vi "Agilent 34970 Temperature Resistance Conversion.vi"(6 "Resistance Value":dbl, 8 "error in (no error)":errorcluster) -> (0 "error out":errorcluster, 4 "Temperature (F)":dbl)   [LabVIEW 2023]
uses:
  <vilib>/Analysis/NI_AALPro.lvlib
panel:
  out "Temperature (C)":dbl
  out "Temperature Array":dbl[](array[numeric])
  out "Resistance Array":dbl[](array[numeric])
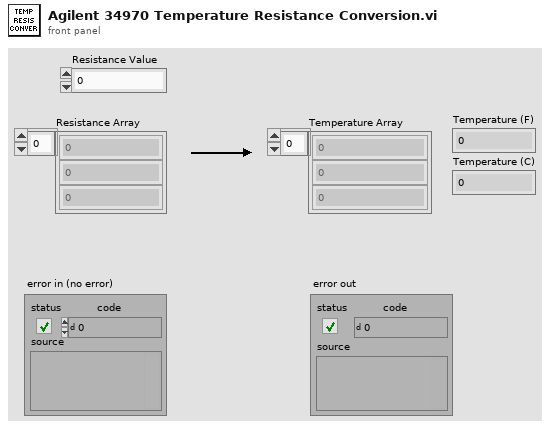
[diagram p1: front panel]
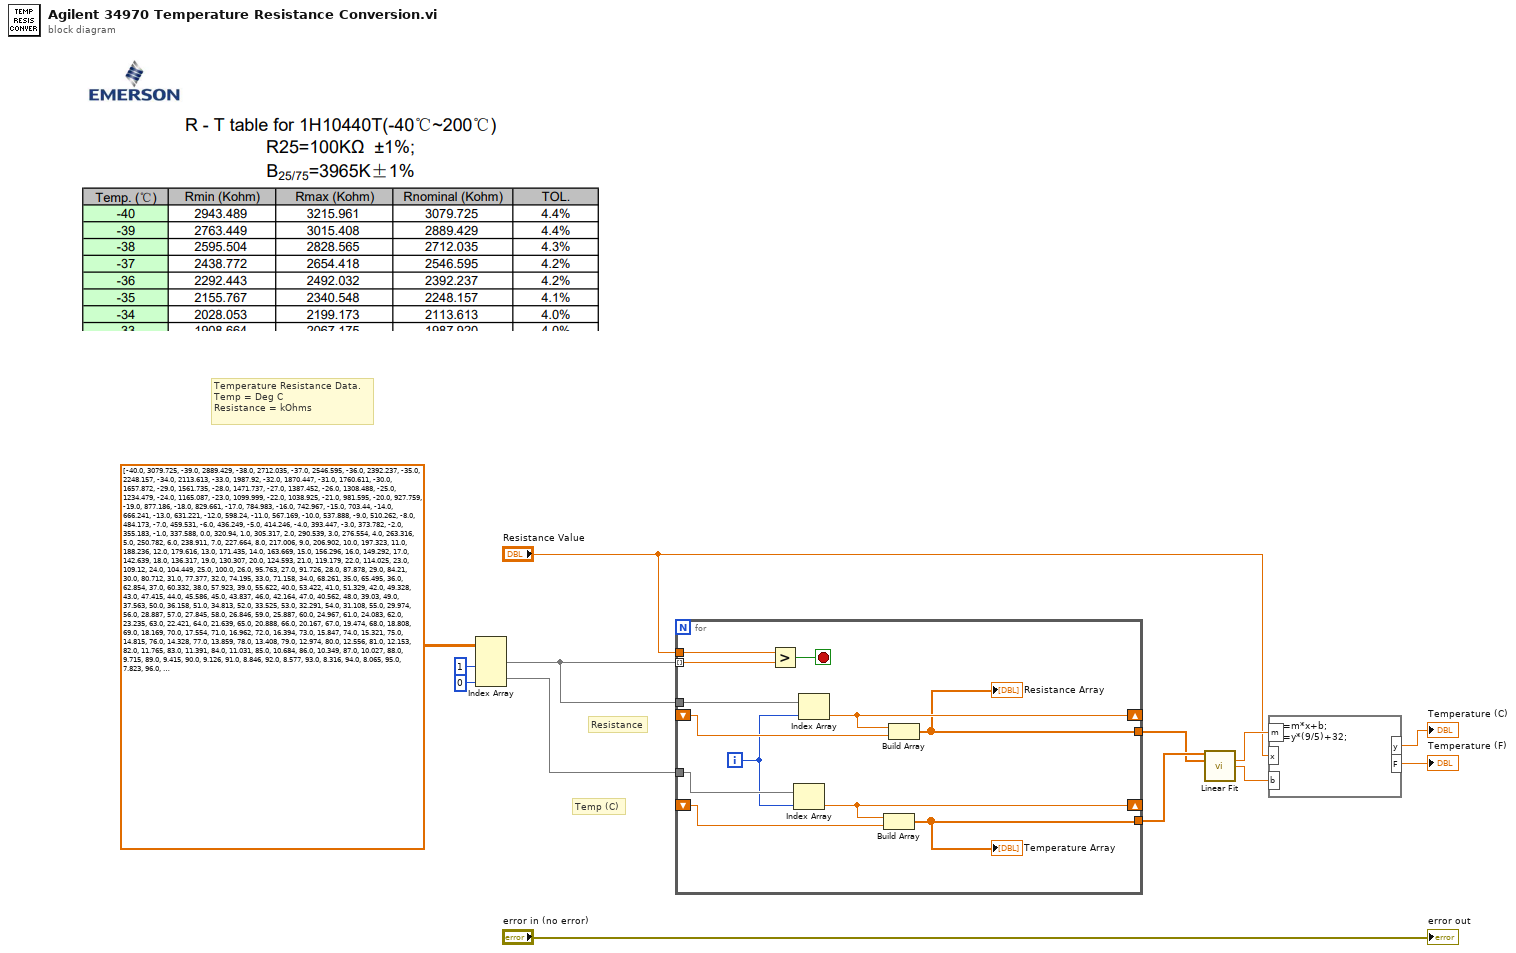
[diagram p0: block diagram]
diagram:
  # "Temp (C)"
  # "Resistance"
  # "Temperature Resistance Data. \nTemp = Deg C\nResistance = kOhms"
  n1 = Index Array(array=dbl[][] [[-40.0, 3079.725], [-39.0, 2889.429], [-38.0, 2712.035], [-37.0, 2546.595], [-36.0, 2392.237], [-35.0, 2248.157], [-34.0, 2113.613], [-33.0, 1987.92], [-32.0, 1870.447], [-31.0, 1760.611], [-30.0, 1657.872], [-29.0, 1561.735], [-28.0, 1471.737], [-27.0, 1387.452], [-26.0, 1308.488], [-25.0, 1234.479], [-24.0, 1165.087], [-23.0, 1099.999], [-22.0, 1038.925], [-21.0, 981.595], [-20.0, 927.759], [-19.0, 877.186], [-18.0, 829.661], [-17.0, 784.983], [-16.0, 742.967], [-15.0, 703.44], [-14.0, 666.241], [-13.0, 631.221], [-12.0, 598.24], [-11.0, 567.169], [-10.0, 537.888], [-9.0, 510.262], [-8.0, 484.173], [-7.0, 459.531], [-6.0, 436.249], [-5.0, 414.246], [-4.0, 393.447], [-3.0, 373.782], [-2.0, 355.183], [-1.0, 337.588], [0.0, 320.94], [1.0, 305.317], [2.0, 290.539], [3.0, 276.554], [4.0, 263.316], [5.0, 250.782], [6.0, 238.911], [7.0, 227.664], [8.0, 217.006], [9.0, 206.902], [10.0, 197.323], [11.0, 188.236], [12.0, 179.616], [13.0, 171.435], [14.0, 163.669], [15.0, 156.296], [16.0, 149.292], [17.0, 142.639], [18.0, 136.317], [19.0, 130.307], [20.0, 124.593], [21.0, 119.179], [22.0, 114.025], [23.0, 109.12], [24.0, 104.449], [25.0, 100.0], [26.0, 95.763], [27.0, 91.726], [28.0, 87.878], [29.0, 84.21], [30.0, 80.712], [31.0, 77.377], [32.0, 74.195], [33.0, 71.158], [34.0, 68.261], [35.0, 65.495], [36.0, 62.854], [37.0, 60.332], [38.0, 57.923], [39.0, 55.622], [40.0, 53.422], [41.0, 51.329], [42.0, 49.328], [43.0, 47.415], [44.0, 45.586], [45.0, 43.837], [46.0, 42.164], [47.0, 40.562], [48.0, 39.03], [49.0, 37.563], [50.0, 36.158], [51.0, 34.813], [52.0, 33.525], [53.0, 32.291], [54.0, 31.108], [55.0, 29.974], [56.0, 28.887], [57.0, 27.845], [58.0, 26.846], [59.0, 25.887], [60.0, 24.967], [61.0, 24.083], [62.0, 23.235], [63.0, 22.421], [64.0, 21.639], [65.0, 20.888], [66.0, 20.167], [67.0, 19.474], [68.0, 18.808], [69.0, 18.169], [70.0, 17.554], [71.0, 16.962], [72.0, 16.394], [73.0, 15.847], [74.0, 15.321], [75.0, 14.815], [76.0, 14.328], [77.0, 13.859], [78.0, 13.408], [79.0, 12.974], [80.0, 12.556], [81.0, 12.153], [82.0, 11.765], [83.0, 11.391], [84.0, 11.031], [85.0, 10.684], [86.0, 10.349], [87.0, 10.027], [88.0, 9.715], [89.0, 9.415], [90.0, 9.126], [91.0, 8.846], [92.0, 8.577], [93.0, 8.316], [94.0, 8.065], [95.0, 7.823], [96.0, 7.589], [97.0, 7.363], [98.0, 7.144], [99.0, 6.933], [100.0, 6.73], [101.0, 6.534], [102.0, 6.344], [103.0, 6.161], [104.0, 5.984], [105.0, 5.812], [106.0, 5.646], [107.0, 5.486], [108.0, 5.331], [109.0, 5.181], [110.0, 5.035], [111.0, 4.894], [112.0, 4.758], [113.0, 4.626], [114.0, 4.499], [115.0, 4.375], [116.0, 4.255], [117.0, 4.139], [118.0, 4.027], [119.0, 3.918], [120.0, 3.812], [121.0, 3.71], [122.0, 3.612], [123.0, 3.516], [124.0, 3.423], [125.0, 3.333], [126.0, 3.246], [127.0, 3.162], [128.0, 3.08], [129.0, 3.0], [130.0, 2.923], [131.0, 2.848], [132.0, 2.775], [133.0, 2.705], [134.0, 2.636], [135.0, 2.57], [136.0, 2.505], [137.0, 2.442], [138.0, 2.382], [139.0, 2.322], [140.0, 2.265], [141.0, 2.209], [142.0, 2.155], [143.0, 2.102], [144.0, 2.051], [145.0, 2.001], [146.0, 1.953], [147.0, 1.906], [148.0, 1.86], [149.0, 1.815], [150.0, 1.772], [151.0, 1.73], [152.0, 1.689], [153.0, 1.65], [154.0, 1.611], [155.0, 1.573], [156.0, 1.537], [157.0, 1.501], [158.0, 1.467], [159.0, 1.433], [160.0, 1.401], [161.0, 1.369], [162.0, 1.338], [163.0, 1.308], [164.0, 1.279], [165.0, 1.25], [166.0, 1.223], [167.0, 1.196], [168.0, 1.169], [169.0, 1.143], [170.0, 1.118], [171.0, 1.094], [172.0, 1.07], [173.0, 1.047], [174.0, 1.024], [175.0, 1.002], [176.0, 0.981], [177.0, 0.96], [178.0, 0.939], [179.0, 0.919], [180.0, 0.9], [181.0, 0.881], [182.0, 0.863], [183.0, 0.845], [184.0, 0.827], [185.0, 0.81], [186.0, 0.793], [187.0, 0.777], [188.0, 0.761], [189.0, 0.746], [190.0, 0.731], [191.0, 0.716], [192.0, 0.701], [193.0, 0.687], [194.0, 0.673], [195.0, 0.66], [196.0, 0.647], [197.0, 0.634], [198.0, 0.621], [199.0, 0.609], [200.0, 0.597]] ("Temp/Resistance Data"), index (col) #1=1 ("disabled index (col)"), index (col) #2=0 ("index (col)")) -> (element #1=w10:dbl[], element #2=w9:dbl[])  [unwired: 2 in]
  n2 = for {
    tunnel: w10 -> [w24] mode=indexing
    tunnel: "Resistance Value" -> [w16]
    tunnel: w10 -> [w23]
    shift-right: [w22] -> _
    shift-left: _ -> [w21]
    tunnel: w9 -> [w20]
    shift-right: [w18] -> _
    shift-left: _ -> [w17]
    tunnel: [w15] -> w3
    tunnel: [w14] -> w4
    i -> [w19]
    stop <- w25 stop-if-true
    n3 = Greater?(x=w16, y=w24) -> (0:w25:bool)
    n4 = Index Array(array=w20, index=w19) -> (element=w18:dbl)
    n5 = Index Array(array=w23, index=w19) -> (element=w22:dbl)
    n6 = Build Array(w18, w17) -> (w14:dbl[])
    "Temperature Array" <- w14
    n7 = Build Array(w22, w21) -> (w15:dbl[])
    "Resistance Array" <- w15
  }
  n8 = call <vilib>:"Linear Fit.vi"("Y"=w4, "X"=w3) -> ("slope"=w7:dbl, "intercept"=w8:dbl)  [unwired: 9 in, 3 out]
  n9 = formula code="y=m*x+b;\nF=y*(9/5)+32;"("m"=w7, "b"=w8, "x"="Resistance Value") -> ("y"=→"Temperature (C)":dbl, "F"=→"Temperature (F)":dbl)
  "error out" <- "error in (no error)"
